vi "Copy Buffer to Image (Custom Stride Greyscale).vi"(7 "Buffer Layout":T2={"Dimension 0"={"Size"=0, "Stride"=0}, "Dimension 1"={"Size"=0, "Stride"=1}}, 8 "error in (no error)":errorcluster, 10 "Greyscale Image Destination in":T1, 11 "Buffer":u8[](array[numeric])) -> (0 "error out":errorcluster, 3 "Greyscale Image Destination":T1)   [LabVIEW 2020, in "image.lvlib"]
doc: "Copy the Buffer into the Image Destination.\n\nThe Destination will be resized to acommodate the Buffer's data."
uses:
  image.lvlib
  f11fe23a-4bac-4ce6-b593-80dfc143e0fd.vi
  Raw Memory Information Dimension.ctl
  Buffer Information.ctl
  Greyscale Image.ctl
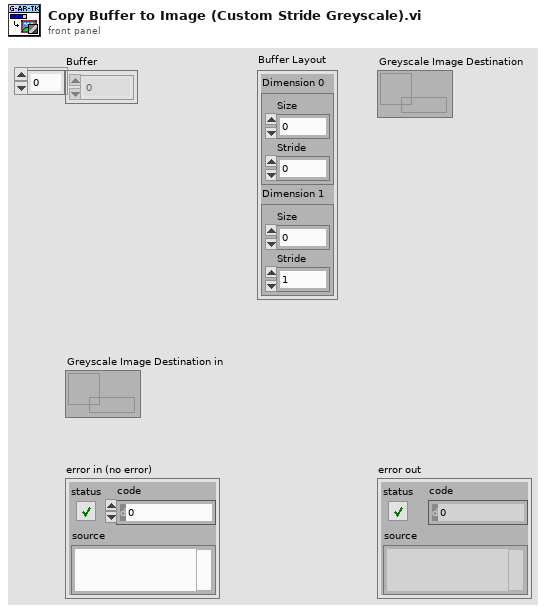
[diagram p1: front panel]
types:
  T1 = typedef "image.lvlib/Greyscale Image.ctl" = refnum<data-value>
  T2 = typedef "image.lvlib/Buffer Information.ctl" = cluster{"Dimension 0":T3, "Dimension 1":T3}
  T3 = typedef "image.lvlib/Raw Memory Information Dimension.ctl" = cluster{"Size":u16, "Stride":i32}
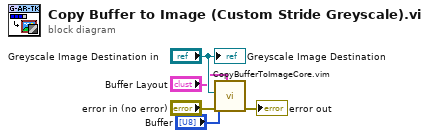
[diagram p0: block diagram]
diagram:
  n1 = call "CopyBufferToImageCore.vim"("Buffer Information"="Buffer Layout", "error in (no error)"="error in (no error)", "Dst"="Greyscale Image Destination in", "Buffer"="Buffer") -> ("error out"=→"error out":errorcluster)  [unwired: 7 in]
  "Greyscale Image Destination" <- "Greyscale Image Destination in"
